vi "Beam Profiler.vi"(7 "Calling VI Ref":refnum<vi>) -> ()   [LabVIEW 2020]
uses:
  Hardware Configuration/Hardware Configuration Controls/Device Type.ctl
  Beam Profiler Controls/Beam Profiler Notifier Type.ctl
  Beam Profiler Controls/Beam Profiler Actions.ctl
  <vilib>/vision/Image Controls.llb/IMAQ Image.ctl
  <vilib>/Utility/miscctls.llb/LVPointTypeDef.ctl
  Device Library/Cameras/Camera Controls/Generic Camera ROI.ctl
  Beam Profiler Controls/Beam Profiler Fit Results.ctl
  Device Library/Cameras/Polymorphic Camera Messenger/Get Status.vi
  Device Library/Cameras/Polymorphic Camera Messenger/Abort.vi
  Device Library/Cameras/Polymorphic Camera Messenger/Set Exp Time.vi
  Device Library/Cameras/Polymorphic Camera Messenger/Get Exp Time.vi
  Device Library/Cameras/Polymorphic Camera Messenger/Set ROI.vi
  Device Library/Cameras/Polymorphic Camera Messenger/Live Preview.vi
  Device Library/Cameras/Polymorphic Camera Messenger/Quit.vi
  <vilib>/vision/NI_Vision_Development_Module.lvlib
panel:
  in  "Setup ROI":bool
  in  "ROI Active":bool
  out "Camera Connected":bool
  in  "Close Camera":bool
  in  "Quit":bool
  out "Y Pos (px)":dbl=1.0 format="%#_4g"
  out "X Pos (px)":dbl=1.0 format="%#_4g"
  out "Y FWHM (mm)":dbl=1.0 format="%#_4g"
  out "Y FWHM (px)":dbl=1.0 format="%#_4g"
  out "X FWHM (mm)":dbl=1.0 format="%#_4g"
  out "X FWHM (px)":dbl=1.0 format="%#_4g"
  in  "Cursor Visible":bool
  in  "Snap Cursor":bool
  in  "Color Map":T1(ring)=enum."Gray"
  out "Fit Image":dbl[][](graph)
  out "Camera Image":u16[][](graph)
  out "Error":bool
  in  "Live Preview":bool
  in  "Exposure Time (ms)":dbl=100.0
  in  "Camera Pixel Size (µm)":dbl=1.0
  in  "Fitting":bool
  in  "Fit Update Rate (ms)":u32=100
  in  "Binning (pixels)":i32=1 min=1 step=1
  in  "Profiler Camera":i32(ring) items=["IDS-Camera-Overview-3"]
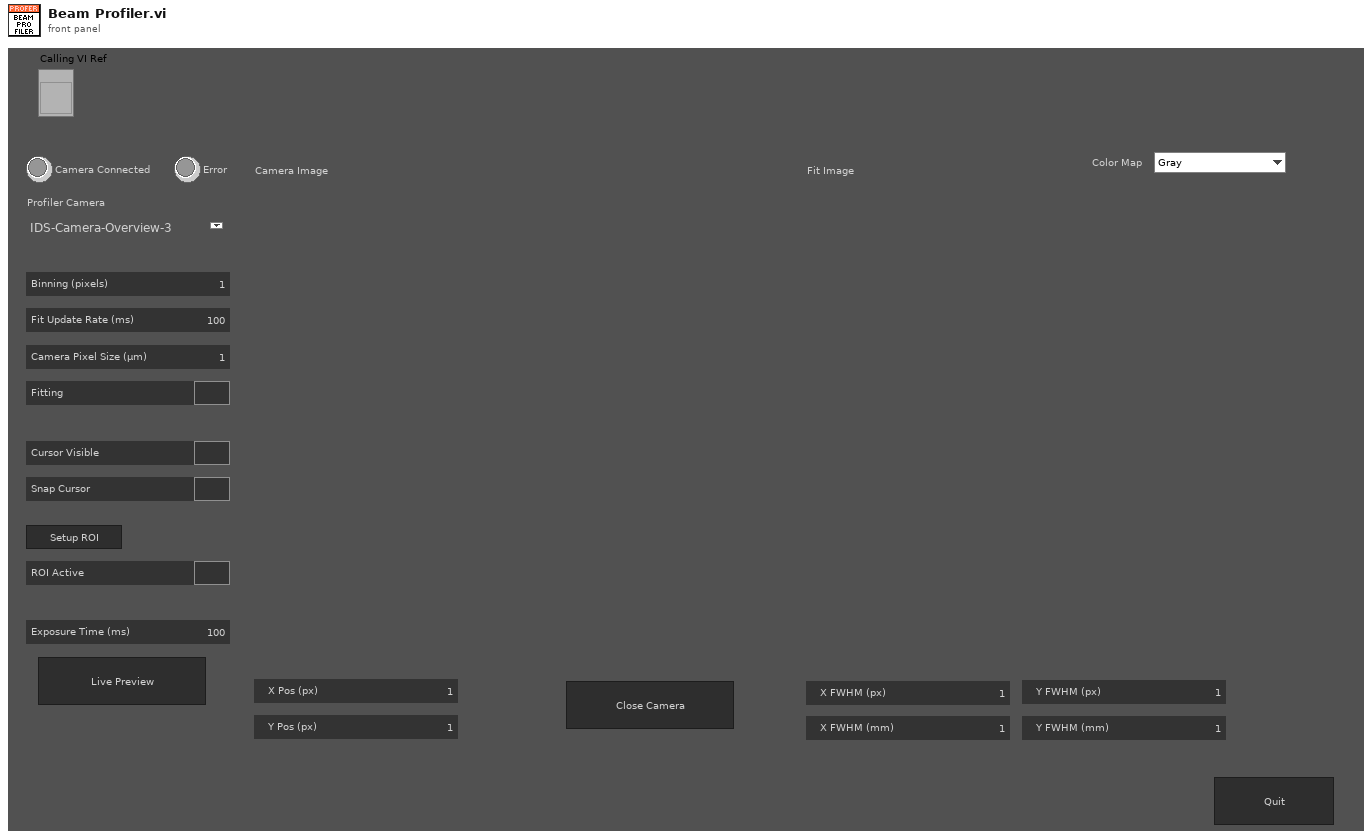
[diagram p1: front panel]
types:
  T1 = enum16{"Fire", "Gray", "Red", "Green", "Blue", "Cyan", "Magenta", "Yellow", "Red-White", "Green-White", "Blue-White", "Glow"}
  T2 = enum16{"Always On", "Always Off", "Off While Running"}
  T3 = typedef "LVPointTypeDef.ctl" = cluster{"Horizontal":i16, "Vertical":i16}
  T4 = typedef "Image Type" = u32
  T5 = typedef "IMAQ Image.ctl" = refnum<image>
  T6 = typedef "Beam Profiler Actions.ctl" = enum16{"Do Nothing", "Switch Camera", "Set Exp Time", "Setup ROI", "ROI Active", "Start Live", "Poll Image", "Stop Camera", "Quit"}
  T7 = typedef "Beam Profiler Notifier Type.ctl" = cluster{"Actions":T6, "Camera Notifier":string, "Pixel Size":dbl, "Binning":i32, "Fitting":bool, "Running?":bool, "Exp Time (ms)":dbl, "Image Ref":T5, "ROI Active":bool}
  T8 = typedef "Device Type.ctl" = enum16{"AOTF", "Camera", "Deformable Mirror", "Laser", "Microscope Base", "Shutter", "Stage", "Waveform", "FPGA", "Email", "Filter Wheel", "Spinning Disk"}
  T9 = typedef "Generic Camera ROI.ctl" = cluster{"H_Offset":u16, "V_Offset":u16, "H_Width":u16, "V_Width":u16}
  T10 = typedef "Beam Profiler Fit Results.ctl" = cluster{"X Position":dbl, "Y Position":dbl, "X FWHM (px)":dbl, "Y FWHM (px)":dbl, "X FWHM (mm)":dbl, "Y FWHM (mm)":dbl}
  T11 = enum8{"Enabled", "Disabled", "Disabled and Grayed Out"}
  T12 = typedef "LVRectTypeDef.ctl" = cluster{"Left":i16, "Top":i16, "Right":i16, "Bottom":i16}
  T13 = typedef "LVBoundsTypeDef.ctl" = cluster{"Width":u32, "Height":u32}
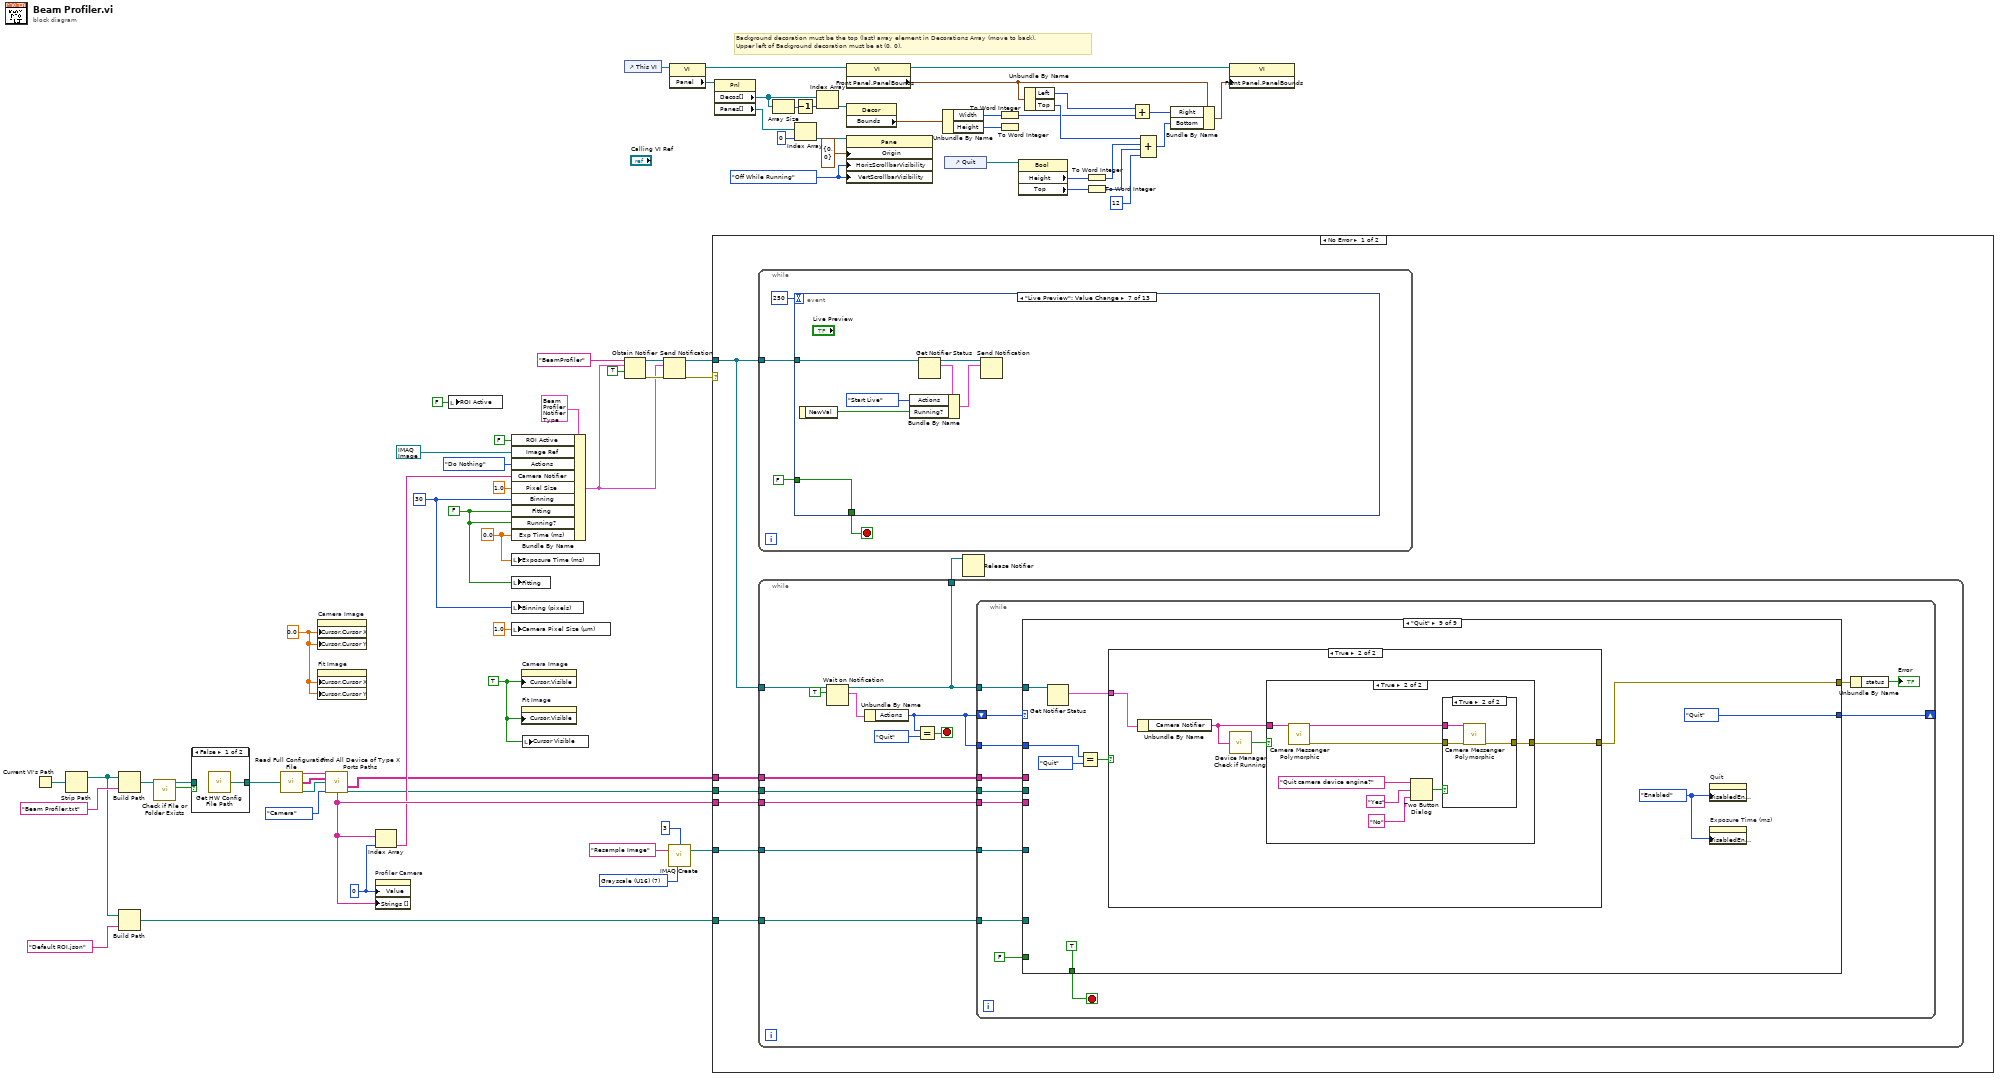
[diagram p0: block diagram]
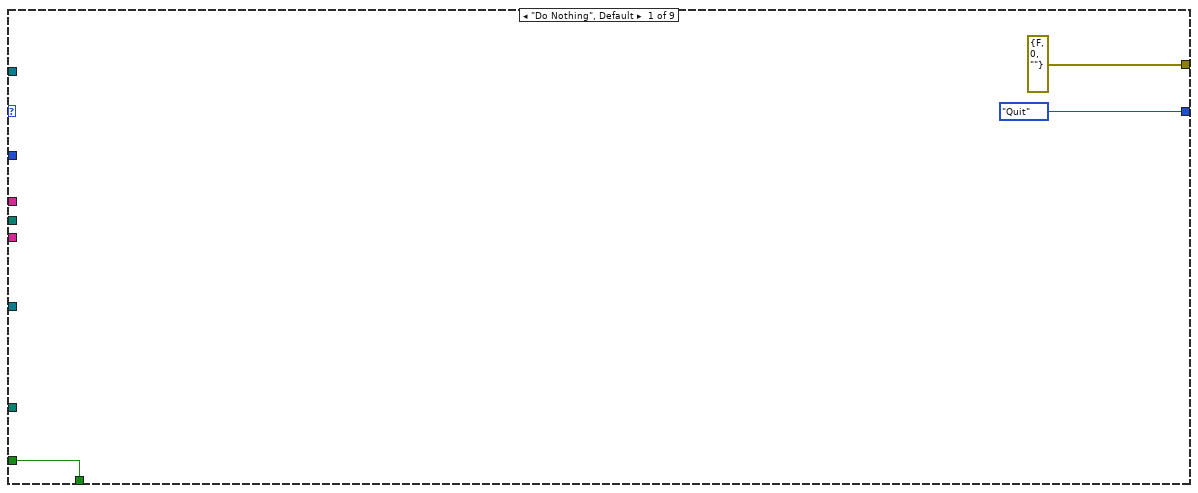
[diagram p3: hidden frame]
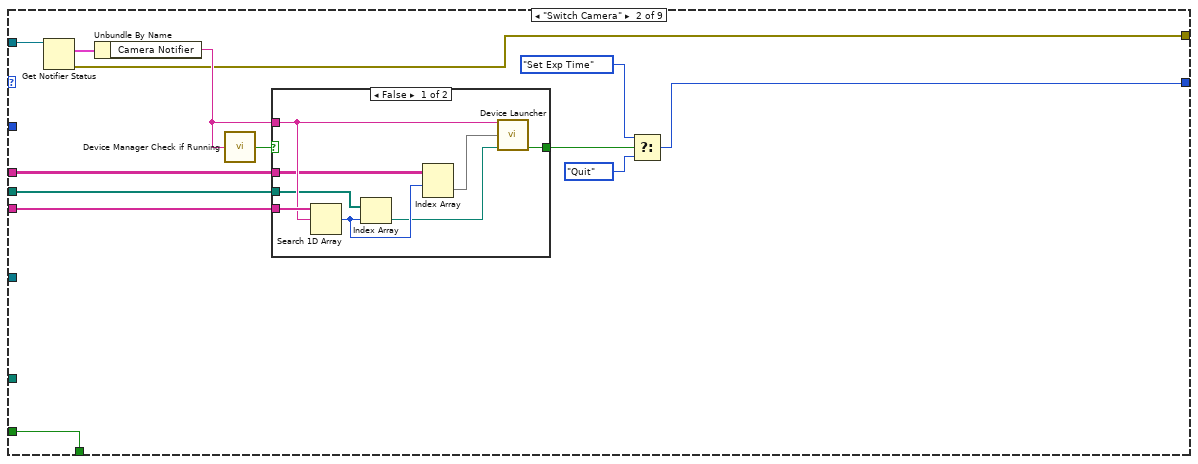
[diagram p4: hidden frame]
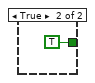
[diagram p5: hidden frame]
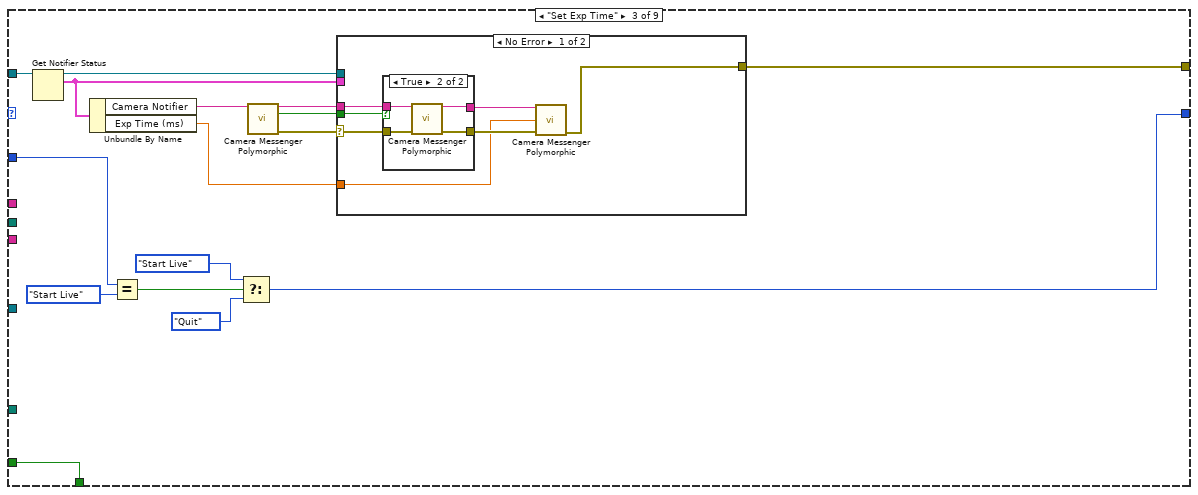
[diagram p6: hidden frame]
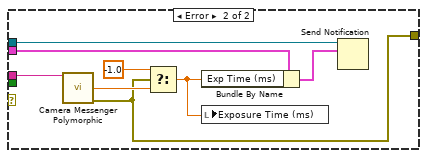
[diagram p8: hidden frame]
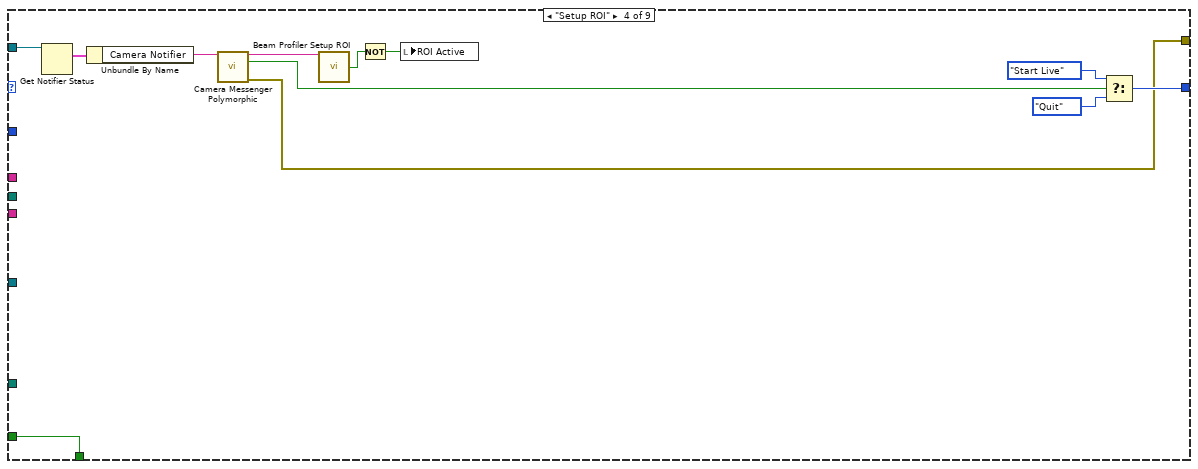
[diagram p9: hidden frame]
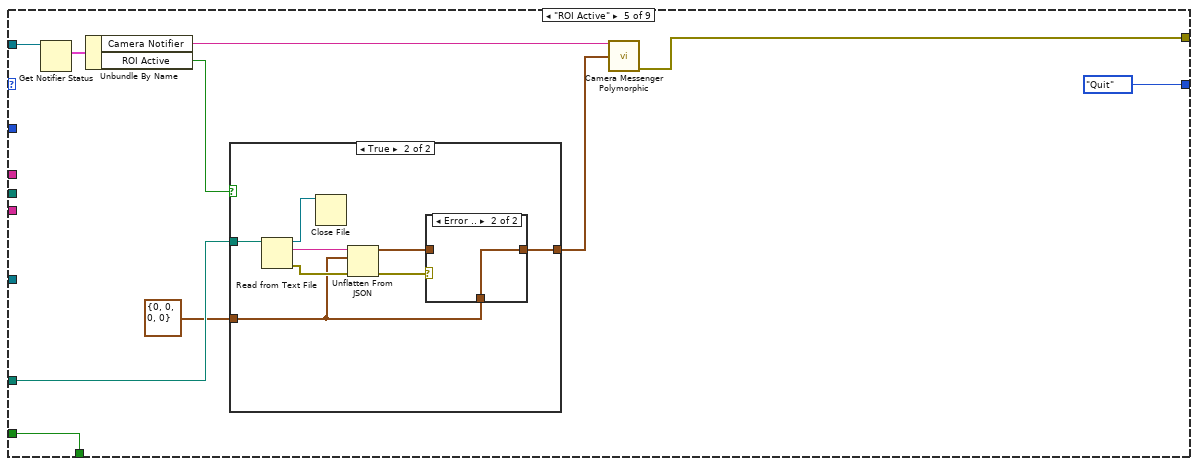
[diagram p10: hidden frame]
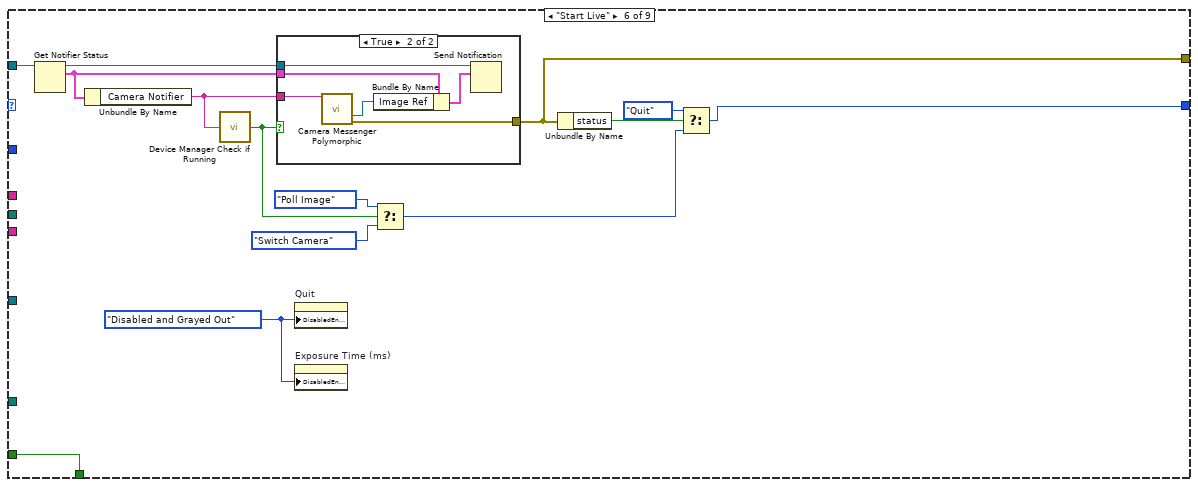
[diagram p13: hidden frame]
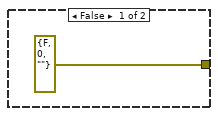
[diagram p14: hidden frame]
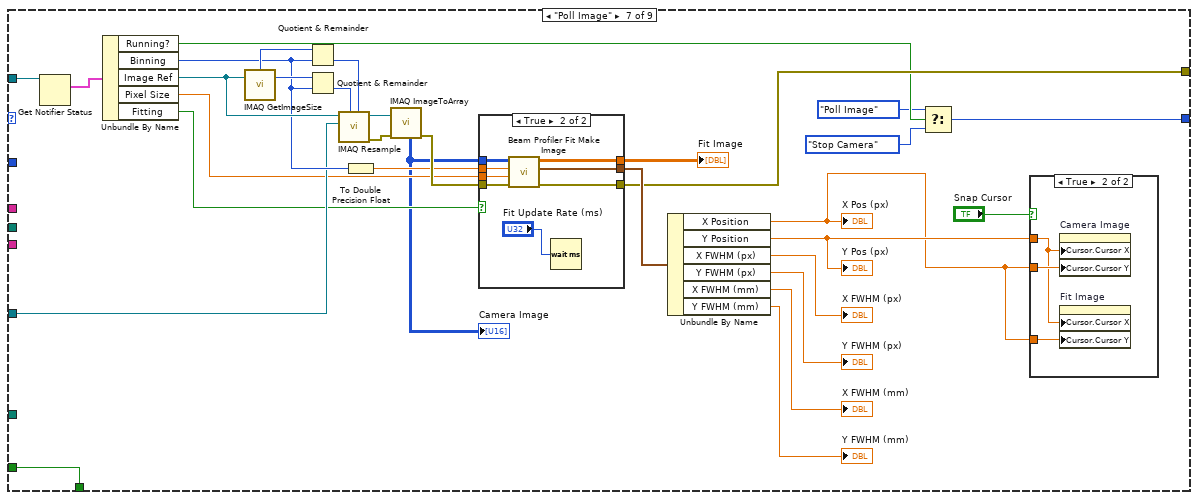
[diagram p15: hidden frame]
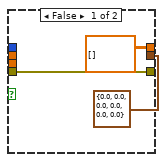
[diagram p17: hidden frame]
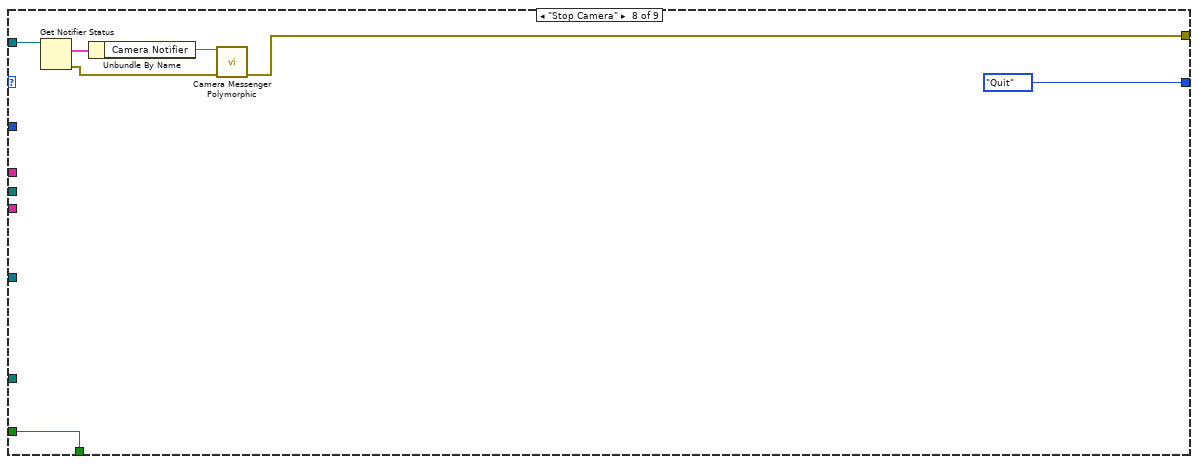
[diagram p18: hidden frame]
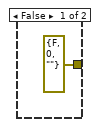
[diagram p19: hidden frame]
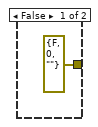
[diagram p20: hidden frame]
diagram:
  w16 = 0.0 ("Cursor.Cursor Position:Cursor X")
  w6 = TRUE ("Cursor.Visible")
  w29 = T2."Off While Running" ("Vertical Scrollbar Visibility")
  w52 = T4 7 items=["Grayscale (U8)", "Grayscale (I16)", "Grayscale (SGL)", "Complex (CSG)", "RGB (U32)", "HSL (U32)", "RGB (U64)", "Grayscale (U16)"] ("Image Type")
  w56 = 0.0 ("Exp Time (sec)")
  w59 = 30 ("Pixel Size")
  w60 = FALSE ("Fitting")
  w54 = 0
  # "Background decoration must be the top (last) array element in Decorations Array (move to back).\nUpper left of Background decoration must be at (0, 0)."
  n1 = Current VI's Path() -> (path=w15:path)
  n2 = Strip Path(path=w15) -> (stripped path=w8:path)  [unwired: 1 out]
  n3 = Build Path(base path=w8, name or relative path="Beam Profiler.txt") -> (appended path=w13:path)
  n4 = Build Path(base path=w8, name or relative path="Default ROI.json") -> (appended path=w7:path)
  n5 = call <vilib>:"Check if File or Folder Exists.vi"("path"=w13) -> ("file or folder exists?"=w12:bool, "dup path"=w11:path)  [unwired: 8 in, 1 out]
  n6 = case shown="False" w12 {
    tunnel: [w71 w72] -> w69
    tunnel: w11 -> [_ w72]
    frame False {
      n7 = call "Get HW Config File Path.vi"() -> ("File Path"=w71:path)  [unwired: 14 in, 1 out]
    }
    frame True {
    }
  }
  n8 = call "Read Full Configuration File.vi"("Config File Path"=w69) -> ("Unique Notifier Names"=w70:string[], "Device Port/ID/Channel Info"=w4:string[][], "Device Engine Paths"=w3:path[])  [unwired: 11 in, 1 out]
  n9 = property on="Camera Image" class="IntGraph (strict)"("Cursor.Cursor X"=w16, "Cursor.Cursor Y"=w16) -> ()  [unwired: 2 in, 2 out]
  n10 = property on="Fit Image" class="IntGraph (strict)"("Cursor.Cursor X"=w16, "Cursor.Cursor Y"=w16) -> ()  [unwired: 2 in, 2 out]
  n11 = call "Find All Device of Type X Ports Paths.vi"("Unique Notifier Names"=w70, "Device Port/ID/Channel Info"=w4, "Device Engine Paths"=w3, "Device Type"=Device_Type."Camera") -> ("All Ports"=w1:string[][], "All Devices"=w55:string[], "All Paths"=w2:path[])  [unwired: 8 in, 1 out]
  n12 = Index Array(array=w55, index=w54) -> (element=w17:string)
  n13 = property on="Profiler Camera" class="Ring (strict)"("Value"=w54, "Strings []"=w55) -> ()  [unwired: 2 in, 2 out]
  n14 = local write "ROI Active"(FALSE ("ROI Active")) -> ()
  n15 = Bundle By Name(cluster=T7 {"Actions"=enum."Do Nothing", "Camera Notifier"="", "Pixel Size"=0.0, "Binning"=0, "Fitting"=FALSE, "Running?"=FALSE, "Exp Time (ms)"=0.0, "Image Ref"=refnum, "ROI Active"=FALSE} ("Beam Profiler Notifier"), "ROI Active"=FALSE, "Image Ref"=T5 refnum, "Actions"=Beam_Profiler_Actions."Do Nothing", "Camera Notifier"=w17, "Pixel Size"=1.0, "Binning"=w59, "Fitting"=w60, "Running?"=w60, "Exp Time (ms)"=w56) -> (w61:T7)
  n16 = local write "Exposure Time (ms)"(w56) -> ()
  n17 = local write "Fitting"(w60) -> ()
  n18 = local write "Binning (pixels)"(w59) -> ()
  n19 = local write "Camera Pixel Size (µm)"(1.0 ("Camera Pixel Size (µm)")) -> ()
  n20 = property on="Camera Image" class="IntGraph (strict)"("Cursor.Visible"=w6) -> ()  [unwired: 2 in, 2 out]
  n21 = property on="Fit Image" class="IntGraph (strict)"("Cursor.Visible"=w6) -> ()  [unwired: 2 in, 2 out]
  n22 = local write "Cursor Visible"(w6) -> ()
  n23 = Obtain Notifier(name (unnamed)="BeamProfiler", notification data type=w61, create if not found? (T)=TRUE) -> (notifier out=w66:refnum<notifier>, error out=w65:errorcluster)  [unwired: 1 in, 1 out]
  n24 = control-ref of="This VI"() -> (w21:refnum<vi>)
  n25 = Send Notification(notification=w61, notifier=w66, error in (no error)=w65) -> (notifier out=w57:refnum<notifier>, error out=w58:errorcluster)
  n26 = call "IMAQ Create"("Border Size"=3, "Image Name"="Resample Image", "Image Type"=w52) -> ("New Image"=w49:T5)  [unwired: 2 in, 1 out]
  n27 = property class="VI"(reference=w21) -> (reference out=w30:refnum<vi>, "Panel"=w22:refnum<vi>)  [unwired: 1 in, 1 out]
  n28 = case shown="No Error" w58 {
    tunnel: w57 -> [w79 _]
    tunnel: w55 -> [w78 _]
    tunnel: w2 -> [w77 _]
    tunnel: w1 -> [w76 _]
    tunnel: w49 -> [w75 _]
    tunnel: w7 -> [w73 _]
    frame No Error {
      n29 = while {
        tunnel: w79 -> [w303]
        stop <- w301 stop-if-true
        n30 = event shown="[6] \"Live Preview\": Value Change" {
          selector: _ -> [_ _ _ _ _ _ _ _ _ _ _ _ _]
          dyn-events: _ -> [_ _ _ _ _ _ _ _ _ _ _ _ _]
          timeout: 250 -> [_ _ _ _ _ _ _ _ _ _ _ _ _]
          tunnel: w303 -> [w310 w319 w333 w338 w345 w352 w359 _ _ w382 w396 w415 w418]
          tunnel: FALSE -> [w311 w323 w336 w343 w350 w357 w364 w366 w369 w387 w406 w416 _]
          tunnel: [w311 w323 w336 w343 w350 w357 w364 w366 w369 w387 w406 w416 TRUE] -> w301
          event Timeout {
            n31 = event-data() -> ()  [unwired: 1 in, 3 out]
            n32 = Get Notifier Status(notifier=w310) -> (current notification=w309:T7)  [unwired: 1 in, 4 out]
            n33 = Unbundle By Name(w309) -> ("Camera Notifier"=w308:string)
            n34 = call "Device Manager Check if Running.vi"("Notifier Name"=w308) -> ("Running?"=w307:bool)  [unwired: 14 in]
            "Camera Connected" <- w307
            n35 = Select(t=T11."Enabled" ("Disabled"), s=w307, f=T11."Disabled and Grayed Out" ("Disabled")) -> (s? t:f=w304:T11)
            n36 = property on="Setup ROI" class="Bool"("DisabledEnum"=w304) -> ()  [unwired: 2 in, 2 out]
            n37 = property on="ROI Active" class="Bool (strict)"("DisabledEnum"=w304) -> ()  [unwired: 2 in, 2 out]
          }
          event "Profiler Camera": Value Change {
            n38 = event-data() -> ("NewVal"=w321:i32, "OldVal"=w314:i32)  [unwired: 1 in]
            n39 = property on="Profiler Camera" class="Ring (strict)"() -> ("Strings []"=w322:string[])  [unwired: 2 in, 2 out]
            n40 = Index Array(array=w322, index #1=w321, index #2=w314) -> (element #1=w317:string, element #2=w313:string)
            n41 = call-poly "Camera Messenger Polymorphic.vi"("Notifier Name"=w313) -> ("Error Out"=w312:errorcluster)  [unwired: 11 in, 3 out]
            n42 = Get Notifier Status(notifier=w319, error in (no error)=w312) -> (notifier out=w320:refnum<notifier>, current notification=w318:T7)  [unwired: 3 out]
            n43 = Bundle By Name(cluster=w318, "Actions"=Beam_Profiler_Actions."Switch Camera", "Camera Notifier"=w317) -> (w316:T7)
            n44 = Send Notification(notification=w316, notifier=w320) -> ()  [unwired: 1 in, 2 out]
          }
          event "Exposure Time (ms)": Value Change {
            n45 = event-data() -> ("NewVal"=w332:dbl)  [unwired: 1 in]
            n46 = Get Notifier Status(notifier=w333) -> (notifier out=w335:refnum<notifier>, current notification=w328:T7)  [unwired: 1 in, 3 out]
            n47 = Divide(x=w332, y=1000.0) -> (x/y=w330:dbl)
            n48 = Unbundle By Name(w328) -> ("Camera Notifier"=w329:string)
            n49 = call "Device Manager Check if Running.vi"("Notifier Name"=w329) -> ("Running?"=w327:bool)  [unwired: 14 in]
            n50 = Select(t=Beam_Profiler_Actions."Set Exp Time" ("Actions"), s=w327, f=Beam_Profiler_Actions."Switch Camera" ("Actions")) -> (s? t:f=w325:T6)
            n51 = Bundle By Name(cluster=w328, "Actions"=w325, "Exp Time (ms)"=w330) -> (w334:T7)
            n52 = Send Notification(notification=w334, notifier=w335) -> ()  [unwired: 1 in, 2 out]
          }
          event "Camera Pixel Size (µm)": Value Change {
            n53 = event-data() -> ("NewVal"=w337:dbl)  [unwired: 1 in]
            n54 = Get Notifier Status(notifier=w338) -> (notifier out=w342:refnum<notifier>, current notification=w341:T7)  [unwired: 1 in, 3 out]
            n55 = Bundle By Name(cluster=w341, "Actions"=Beam_Profiler_Actions."Do Nothing", "Pixel Size"=w337) -> (w340:T7)
            n56 = Send Notification(notification=w340, notifier=w342) -> ()  [unwired: 1 in, 2 out]
          }
          event "Binning (pixels)": Value Change {
            n57 = event-data() -> ("NewVal"=w344:i32)  [unwired: 1 in]
            n58 = Get Notifier Status(notifier=w345) -> (notifier out=w349:refnum<notifier>, current notification=w348:T7)  [unwired: 1 in, 3 out]
            n59 = Bundle By Name(cluster=w348, "Actions"=Beam_Profiler_Actions."Do Nothing", "Binning"=w344) -> (w347:T7)
            n60 = Send Notification(notification=w347, notifier=w349) -> ()  [unwired: 1 in, 2 out]
          }
          event "Fitting": Value Change {
            n61 = event-data() -> ("NewVal"=w351:bool)  [unwired: 1 in]
            n62 = Get Notifier Status(notifier=w352) -> (notifier out=w356:refnum<notifier>, current notification=w355:T7)  [unwired: 1 in, 3 out]
            n63 = Bundle By Name(cluster=w355, "Actions"=Beam_Profiler_Actions."Do Nothing", "Fitting"=w351) -> (w354:T7)
            n64 = Send Notification(notification=w354, notifier=w356) -> ()  [unwired: 1 in, 2 out]
          }
          event "Live Preview": Value Change {
            n65 = event-data() -> ("NewVal"=w358:bool)  [unwired: 1 in]
            n66 = Get Notifier Status(notifier=w359) -> (notifier out=w363:refnum<notifier>, current notification=w362:T7)  [unwired: 1 in, 3 out]
            n67 = Bundle By Name(cluster=w362, "Actions"=Beam_Profiler_Actions."Start Live", "Running?"=w358) -> (w361:T7)
            n68 = Send Notification(notification=w361, notifier=w363) -> ()  [unwired: 1 in, 2 out]
          }
          event "Cursor Visible": Value Change {
            n69 = event-data() -> ("NewVal"=w365:bool)  [unwired: 1 in]
            n70 = property on="Camera Image" class="IntGraph (strict)"("Cursor.Visible"=w365) -> ()  [unwired: 2 in, 2 out]
            n71 = property on="Fit Image" class="IntGraph (strict)"("Cursor.Visible"=w365) -> ()  [unwired: 2 in, 2 out]
          }
          event "Color Map": Value Change {
            n72 = event-data() -> ("NewVal"=w368:T1)  [unwired: 1 in]
            n73 = case shown="\"Fire\", Default" w368 {
              tunnel: [cluster{dbl, u32}[] [{0.0, 0}, {85.0, 16711680}, {108.0, 16729344}, {127.0, 16744192}, {132.0, 16747520}, {140.0, 16753920}, {157.0, 16766720}, {170.0, 16776960}, {245.0, 16777184}, {250.0, 16777200}, {255.0, 16777215}] ("Z Scale.Marker Values[]") cluster{dbl, u32}[] [{0.0, 0}, {255.0, 16777215}] ("Z Scale.Marker Values[]") cluster{dbl, u32}[] [{0.0, 0}, {255.0, 16711680}] ("Z Scale.Marker Values[]") cluster{dbl, u32}[] [{0.0, 0}, {255.0, 65280}] ("Z Scale.Marker Values[]") cluster{dbl, u32}[] [{0.0, 0}, {255.0, 255}] ("Z Scale.Marker Values[]") cluster{dbl, u32}[] [{0.0, 0}, {255.0, 65535}] ("Z Scale.Marker Values[]") cluster{dbl, u32}[] [{0.0, 0}, {255.0, 16711935}] ("Z Scale.Marker Values[]") cluster{dbl, u32}[] [{0.0, 0}, {255.0, 16776960}] ("Z Scale.Marker Values[]") cluster{dbl, u32}[] [{0.0, 0}, {170.0, 16711680}, {245.0, 16777184}, {250.0, 16777200}, {255.0, 16448250}] ("Z Scale.Marker Values[]") cluster{dbl, u32}[] [{0.0, 0}, {170.0, 65280}, {245.0, 16777184}, {250.0, 16777200}, {255.0, 16448250}] ("Z Scale.Marker Values[]") cluster{dbl, u32}[] [{0.0, 0}, {170.0, 255}, {245.0, 16777184}, {250.0, 16777200}, {255.0, 16448250}] ("Z Scale.Marker Values[]") cluster{dbl, u32}[] [{0.0, 0}, {1.0, 131072}, {2.0, 196608}, {3.0, 327680}, {4.0, 458752}, {5.0, 589824}, {6.0, 720896}, {7.0, 851971}, {8.0, 983043}, {9.0, 1114115}, {10.0, 1245187}, {11.0, 1376259}, {12.0, 1507331}, {13.0, 1638403}, {14.0, 1769475}, {15.0, 1769479}, {16.0, 2031623}, {17.0, 2162695}, {18.0, 2293767}, {19.0, 2424839}, {20.0, 2555911}, {21.0, 2686983}, {22.0, 2818055}, {23.0, 2949127}, {24.0, 3080203}, {25.0, 3211275}, {26.0, 3342347}, {27.0, 3473419}, {28.0, 3604491}, {29.0, 3735563}, {30.0, 3866635}, {31.0, 3867403}, {32.0, 4129547}, {33.0, 4260619}, {34.0, 4391691}, {35.0, 4522763}, {36.0, 4653839}, {37.0, 4784911}, {38.0, 4915983}, {39.0, 5178127}, {40.0, 5309199}, {41.0, 5440271}, {42.0, 5571343}, {43.0, 5702415}, {44.0, 5703439}, {45.0, 5965583}, {46.0, 6096655}, {47.0, 6227727}, {48.0, 6358799}, {49.0, 6489871}, {50.0, 6620943}, {51.0, 6752015}, {52.0, 6883087}, {53.0, 7015183}, {54.0, 7146255}, {55.0, 7277327}, {56.0, 7408399}, {57.0, 7539471}, {58.0, 7670543}, {59.0, 7801615}, {60.0, 8063759}, {61.0, 8194831}, {62.0, 8326927}, {63.0, 8457999}, {64.0, 8589075}, {65.0, 8720147}, {66.0, 8851219}, {67.0, 8982291}, {68.0, 9113363}, {69.0, 9114387}, {70.0, 9376531}, {71.0, 9507603}, {72.0, 9638675}, {73.0, 9769747}, {74.0, 9901843}, {75.0, 10032915}, {76.0, 10163987}, {77.0, 10229523}, {78.0, 10295059}, {79.0, 10427155}, {80.0, 10558227}, {81.0, 10689299}, {82.0, 10820371}, {83.0, 10886931}, {84.0, 10952467}, {85.0, 11083539}, {86.0, 11214611}, {87.0, 11215635}, {88.0, 11477779}, {89.0, 11543315}, {90.0, 11608851}, {91.0, 11740947}, {92.0, 11806483}, {93.0, 11872019}, {94.0, 12004115}, {95.0, 12135187}, {96.0, 12266259}, {97.0, 12267283}, {98.0, 12398355}, {99.0, 12529427}, {100.0, 12530451}, {101.0, 12595987}, {102.0, 12530451}, {103.0, 12793619}, {104.0, 12794131}, {105.0, 12794643}, {106.0, 13056787}, {107.0, 13057299}, {108.0, 13057811}, {109.0, 13188883}, {110.0, 13320979}, {111.0, 13386515}, {112.0, 13452563}, {113.0, 13584147}, {114.0, 13584659}, {115.0, 13585171}, {116.0, 13585683}, {117.0, 13717267}, {118.0, 13848339}, {119.0, 13849363}, {120.0, 13849875}, {121.0, 13850387}, {122.0, 13981459}, {123.0, 14113555}, {124.0, 14114067}, {125.0, 14114579}, {126.0, 14115091}, {127.0, 14246675}, {128.0, 14377747}, {129.0, 14378771}, {130.0, 14379283}, {131.0, 14379539}, {132.0, 14379795}, {133.0, 14380819}, {134.0, 14511891}, {135.0, 14643987}, {136.0, 14644503}, {137.0, 14645015}, {138.0, 14645527}, {139.0, 14646039}, {140.0, 14646551}, {141.0, 14778135}, {142.0, 14909207}, {143.0, 14910231}, {144.0, 14910747}, {145.0, 14911259}, {146.0, 14911771}, {147.0, 14912283}, {148.0, 14912797}, {149.0, 15044383}, {150.0, 15175455}, {151.0, 15175967}, {152.0, 15176479}, {153.0, 15176991}, {154.0, 15177507}, {155.0, 15178019}, {156.0, 15178531}, {157.0, 15310115}, {158.0, 15441701}, {159.0, 15441959}, {160.0, 15442215}, {161.0, 15442727}, {162.0, 15443243}, {163.0, 15443755}, {164.0, 15444269}, {165.0, 15444783}, {166.0, 15444783}, {167.0, 15576367}, {168.0, 15707953}, {169.0, 15708467}, {170.0, 15708979}, {171.0, 15708981}, {172.0, 15708983}, {173.0, 15710011}, {174.0, 15710523}, {175.0, 15711037}, {176.0, 15711039}, {177.0, 15711553}, {178.0, 15843139}, {179.0, 15974213}, {180.0, 15974215}, {181.0, 15974217}, {182.0, 15974219}, {183.0, 15975755}, {184.0, 15976271}, {185.0, 15976785}, {186.0, 15977299}, {187.0, 15977301}, {188.0, 15977815}, {189.0, 15978327}, {190.0, 15978331}, {191.0, 16109917}, {192.0, 16241503}, {193.0, 16241505}, {194.0, 16242019}, {195.0, 16242535}, {196.0, 16242537}, {197.0, 16242539}, {198.0, 16243563}, {199.0, 16243567}, {200.0, 16244081}, {201.0, 16244595}, {202.0, 16244599}, {203.0, 16244601}, {204.0, 16244603}, {205.0, 16245627}, {206.0, 16245631}, {207.0, 16245633}, {208.0, 16246147}, {209.0, 16246663}, {210.0, 16377735}, {211.0, 16508811}, {212.0, 16508815}, {213.0, 16509839}, {214.0, 16509843}, {215.0, 16509845}, {216.0, 16509847}, {217.0, 16510361}, {218.0, 16510875}, {219.0, 16510879}, {220.0, 16510881}, {221.0, 16510883}, {222.0, 16511399}, {223.0, 16511911}, {224.0, 16511915}, {225.0, 16511917}, {226.0, 16511919}, {227.0, 16511923}, {228.0, 16512437}, {229.0, 16512951}, {230.0, 16512955}, {231.0, 16512957}, {232.0, 16512959}, {233.0, 16512961}, {234.0, 16512963}, {235.0, 16512967}, {236.0, 16513481}, {237.0, 16513995}, {238.0, 16513999}, {239.0, 16514001}, {240.0, 16514003}, {241.0, 16514005}, {242.0, 16514007}, {243.0, 16514011}, {244.0, 16514013}, {245.0, 16514015}, {246.0, 16514019}, {247.0, 16514021}, {248.0, 16514023}, {249.0, 16514027}, {250.0, 16514029}, {251.0, 16514031}, {252.0, 16514035}, {253.0, 16514037}, {254.0, 16514039}, {255.0, 16514043}] ("Z Scale.Marker Values[]")] -> w367
              frame "Fire", Default {
                # "Fire"
              }
              frame "Gray" {
                # "Grayscale"
              }
              frame "Red" {
                # "Red"
              }
              frame "Green" {
                # "Green"
              }
              frame "Blue" {
                # "Blue"
              }
              frame "Cyan" {
                # "Cyan"
              }
              frame "Magenta" {
                # "Magenta"
              }
              frame "Yellow" {
                # "Yellow"
              }
              frame "Red-White" {
                # "Red-White"
              }
              frame "Green-White" {
                # "Green-White"
              }
              frame "Blue-White" {
                # "Blue-White"
              }
              frame "Glow" {
              }
            }
            n74 = property on="Camera Image" class="IntGraph (strict)"("ZScale.MarkerVals[]"=w367) -> ()  [unwired: 2 in, 2 out]
            n75 = property on="Fit Image" class="IntGraph (strict)"("ZScale.MarkerVals[]"=w367) -> ()  [unwired: 2 in, 2 out]
          }
          event "Setup ROI": Value Change {
            n76 = event-data() -> ()  [unwired: 1 in, 1 out]
            n77 = Get Notifier Status(notifier=w382) -> (notifier out=w386:refnum<notifier>, current notification=w385:T7)  [unwired: 1 in, 3 out]
            n78 = Bundle By Name(cluster=w385, "Actions"=Beam_Profiler_Actions."Setup ROI") -> (w384:T7)
            n79 = Send Notification(notification=w384, notifier=w386) -> ()  [unwired: 1 in, 2 out]
          }
          event "ROI Active": Value Change {
            n80 = event-data() -> ("NewVal"=w401:bool)  [unwired: 1 in]
            n81 = Get Notifier Status(notifier=w396) -> (notifier out=w398:refnum<notifier>, current notification=w399:T7, error out=w393:errorcluster)  [unwired: 1 in, 2 out]
            n82 = Bundle By Name(cluster=w399, "Actions"=Beam_Profiler_Actions."Do Nothing", "Running?"=FALSE) -> (w400:T7)
            n83 = Send Notification(notification=w400, notifier=w398, error in (no error)=w393) -> (notifier out=w394:refnum<notifier>, error out=w392:errorcluster)
            n84 = local write "Live Preview"(FALSE ("Live Preview")) -> ()
            n85 = while {
              tunnel: w394 -> [w412]
              tunnel: w392 -> [w411]
              tunnel: [w408] -> w391
              tunnel: [w407] -> w390
              stop <- w409 stop-if-true
              n86 = Get Notifier Status(notifier=w412, error in (no error)=w411) -> (notifier out=w408:refnum<notifier>, # waiting=w410:i32, error out=w407:errorcluster)  [unwired: 2 out]
              n87 = Greater Than 0?(x=w410) -> (x > 0?=w409:bool)
            }
            n88 = Get Notifier Status(notifier=w391, error in (no error)=w390) -> (notifier out=w405:refnum<notifier>, current notification=w404:T7, error out=w389:errorcluster)  [unwired: 2 out]
            n89 = Bundle By Name(cluster=w404, "Actions"=Beam_Profiler_Actions."ROI Active", "ROI Active"=w401) -> (w403:T7)
            n90 = Send Notification(notification=w403, notifier=w405, error in (no error)=w389) -> ()  [unwired: 2 out]
          }
          event "Close Camera": Value Change {
            n91 = event-data() -> ()  [unwired: 1 in, 1 out]
            n92 = Get Notifier Status(notifier=w415) -> (current notification=w414:T7)  [unwired: 1 in, 4 out]
            n93 = Unbundle By Name(w414) -> ("Camera Notifier"=w413:string)
            n94 = call-poly "Camera Messenger Polymorphic.vi"("Notifier Name"=w413) -> ()  [unwired: 13 in, 2 out]
          }
          event "Quit": Value Change {
            n95 = event-data() -> ()  [unwired: 1 in, 1 out]
            n96 = Get Notifier Status(notifier=w418) -> (notifier out=w422:refnum<notifier>, current notification=w421:T7)  [unwired: 1 in, 3 out]
            n97 = Bundle By Name(cluster=w421, "Actions"=Beam_Profiler_Actions."Quit") -> (w420:T7)
            n98 = Send Notification(notification=w420, notifier=w422) -> ()  [unwired: 1 in, 2 out]
          }
        }
      }
      n99 = while {
        tunnel: w79 -> [w91]
        tunnel: w78 -> [w87]
        tunnel: w77 -> [w86]
        tunnel: w76 -> [w85]
        tunnel: w75 -> [w83]
        tunnel: [w82] -> w74
        tunnel: w73 -> [w80]
        stop <- w88 stop-if-true
        n100 = Wait on Notification(notifier=w91, ignore previous (F)=TRUE) -> (notifier out=w82:refnum<notifier>, notification=w90:T7)  [unwired: 2 in, 2 out]
        n101 = Unbundle By Name(w90) -> ("Actions"=w84:T6)
        n102 = Equal?(x=w84, y=Beam_Profiler_Actions."Quit") -> (x = y?=w88:bool)
        n103 = while {
          tunnel: w82 -> [w103]
          tunnel: w87 -> [w100]
          tunnel: w86 -> [w99]
          tunnel: w85 -> [w98]
          shift-right: [w97] -> _
          shift-left: w84 -> [w104]
          tunnel: w84 -> [w96]
          tunnel: w83 -> [w95]
          tunnel: w80 -> [w92]
          stop <- w101 stop-if-true
          n104 = case shown="\"Quit\"" w104 {
            tunnel: w103 -> [_ w119 w145 w174 w187 w212 w250 w271 w277]
            tunnel: FALSE -> [w107 w120 w144 w178 w186 w213 w251 w270 _]
            tunnel: [w107 w120 w144 w178 w186 w213 w251 w270 TRUE] -> w101
            tunnel: w100 -> [_ w113 _ _ _ _ _ _ _]
            tunnel: w99 -> [_ w115 _ _ _ _ _ _ _]
            tunnel: w98 -> [_ w114 _ _ _ _ _ _ _]
            tunnel: [Beam_Profiler_Actions."Quit" ("f") w109 w133 w168 Beam_Profiler_Actions."Quit" ("f") w205 w225 Beam_Profiler_Actions."Quit" ("f") Beam_Profiler_Actions."Quit" ("f")] -> w97
            tunnel: [errorcluster {"status"=FALSE, "code"=0, "source"=""} ("Error Out") w108 w142 w167 w181 w208 w229 w267 w274] -> w93
            tunnel: w96 -> [_ _ w140 _ _ _ _ _ w278]
            tunnel: w95 -> [_ _ _ _ _ _ w240 _ _]
            tunnel: w92 -> [_ _ _ _ w184 _ _ _ _]
            frame "Do Nothing", Default {
            }
            frame "Switch Camera" {
              n105 = Get Notifier Status(notifier=w119) -> (current notification=w118:T7, error out=w108:errorcluster)  [unwired: 1 in, 3 out]
              n106 = Unbundle By Name(w118) -> ("Camera Notifier"=w116:string)
              n107 = call "Device Manager Check if Running.vi"("Notifier Name"=w116) -> ("Running?"=w117:bool)  [unwired: 14 in]
              n108 = case shown="False" w117 {
                tunnel: w116 -> [w127 _]
                tunnel: w115 -> [w125 _]
                tunnel: w114 -> [w126 _]
                tunnel: w113 -> [w128 _]
                tunnel: [w121 TRUE ("Running?")] -> w112
                frame False {
                  n109 = Search 1D Array(1D array=w128, element=w127) -> (index of element=w124:i32)  [unwired: 1 in]
                  n110 = Index Array(array=w125, index=w124) -> (element=w122:path)
                  n111 = Index Array(array=w126, index (row)=w124) -> (element=w123:string[])  [unwired: 1 in]
                  n112 = call "Device Launcher.vi"("Notifier Name"=w127, "Device Ports/IDs/Channels"=w123, "Device Engine Path"=w122) -> ("Running?"=w121:bool)  [unwired: 11 in, 1 out]
                }
                frame True {
                }
              }
              n113 = Select(t=Beam_Profiler_Actions."Set Exp Time" ("y"), s=w112, f=Beam_Profiler_Actions."Quit" ("y")) -> (s? t:f=w109:T6)
            }
            frame "Set Exp Time" {
              n114 = Get Notifier Status(notifier=w145) -> (notifier out=w136:refnum<notifier>, current notification=w135:T7)  [unwired: 1 in, 3 out]
              n115 = Unbundle By Name(w135) -> ("Camera Notifier"=w134:string, "Exp Time (ms)"=w143:dbl)
              n116 = Equal?(x=w140, y=Beam_Profiler_Actions."Start Live" ("x")) -> (x = y?=w139:bool)
              n117 = Select(t=Beam_Profiler_Actions."Start Live", s=w139, f=Beam_Profiler_Actions."Quit" ("y")) -> (s? t:f=w133:T6)
              n118 = call-poly "Camera Messenger Polymorphic.vi"("Notifier Name"=w134) -> ("Notifier Name DUP"=w131:string, "Running?"=w132:bool, "Error Out"=w130:errorcluster)  [unwired: 10 in, 2 out]
              n119 = case shown="No Error" w130 {
                selector: w130 -> [w146 _]
                tunnel: w132 -> [w152 _]
                tunnel: w131 -> [w151 w166]
                tunnel: w143 -> [w148 _]
                tunnel: [w147 w160] -> w142
                tunnel: w136 -> [_ w165]
                tunnel: w135 -> [_ w164]
                frame No Error {
                  n120 = case shown="True" w152 {
                    tunnel: w151 -> [w154 w158]
                    tunnel: w146 -> [w153 w157]
                    tunnel: [w154 w156] -> w150
                    tunnel: [w153 w155] -> w149
                    frame False {
                    }
                    frame True {
                      n121 = call-poly "Camera Messenger Polymorphic.vi"("Notifier Name"=w158, "Error In"=w157) -> ("Notifier Name DUP"=w156:string, "Error Out"=w155:errorcluster)  [unwired: 10 in, 2 out]
                    }
                  }
                  n122 = call-poly "Camera Messenger Polymorphic.vi"("Notifier Name"=w150, "Exp Time (s)"=w148, "Error In"=w149) -> ("Error Out"=w147:errorcluster)  [unwired: 9 in, 3 out]
                }
                frame Error {
                  n123 = call-poly "Camera Messenger Polymorphic.vi"("Notifier Name"=w166) -> ("Exp Time (s)"=w162:dbl, "Error Out"=w160:errorcluster)  [unwired: 12 in, 1 out]
                  n124 = Select(t=-1.0, s=w160, f=w162) -> (s? t:f=w159:dbl)
                  n125 = Bundle By Name(cluster=w164, "Exp Time (ms)"=w159) -> (w163:T7)
                  n126 = local write "Exposure Time (ms)"(w159) -> ()
                  n127 = Send Notification(notification=w163, notifier=w165) -> ()  [unwired: 1 in, 2 out]
                }
              }
            }
            frame "Setup ROI" {
              n128 = Get Notifier Status(notifier=w174) -> (current notification=w175:T7)  [unwired: 1 in, 4 out]
              n129 = Unbundle By Name(w175) -> ("Camera Notifier"=w173:string)
              n130 = call-poly "Camera Messenger Polymorphic.vi"("Notifier Name"=w173) -> ("Notifier Name DUP"=w172:string, "Running?"=w169:bool, "Error Out"=w167:errorcluster)  [unwired: 10 in, 2 out]
              n131 = call "Beam Profiler Setup ROI.vi"("Camera Notifier Name"=w172) -> ("Canceled?"=w177:bool)  [unwired: 14 in]
              n132 = Not(x=w177) -> (.not. x?=w176:bool)
              n133 = local write "ROI Active"(w176) -> ()
              n134 = Select(t=Beam_Profiler_Actions."Start Live" ("f"), s=w169, f=Beam_Profiler_Actions."Quit") -> (s? t:f=w168:T6)
            }
            frame "ROI Active" {
              n135 = Get Notifier Status(notifier=w187) -> (current notification=w188:T7)  [unwired: 1 in, 4 out]
              n136 = Unbundle By Name(w188) -> ("Camera Notifier"=w180:string, "ROI Active"=w185:bool)
              n137 = case shown="True" w185 {
                tunnel: w184 -> [_ w197]
                tunnel: [w189 w191] -> w182
                tunnel: T9 {"H_Offset"=0, "V_Offset"=0, "H_Width"=0, "V_Width"=0} ("General_Camera_ROI") -> [w189 w190]
                frame False {
                }
                frame True {
                  n138 = Read from Text File(file (use dialog)=w197) -> (refnum out=w195:refnum<file>, text=w196:string, error out=w194:errorcluster)  [unwired: 3 in, 1 out]
                  n139 = Close File(refnum=w195) -> ()  [unwired: 1 in, 2 out]
                  n140 = Unflatten From JSON(JSON string=w196, type and defaults=w190, error in (no error)=w194) -> (value=w192:T9, error out=w193:errorcluster)  [unwired: 4 in]
                  n141 = case shown="Error .." w193 {
                    tunnel: w192 -> [w198 _]
                    tunnel: [w198 w199] -> w191
                    tunnel: w190 -> [_ w199]
                    frame No Error {
                    }
                    frame Error {
                    }
                  }
                }
              }
              n142 = call-poly "Camera Messenger Polymorphic.vi"("Notifier Name"=w180, "Camera ROI"=w182) -> ("Error Out"=w181:errorcluster)  [unwired: 12 in, 1 out]
            }
            frame "Start Live" {
              w200 = T11."Disabled and Grayed Out" ("Disabled")
              n143 = Get Notifier Status(notifier=w212) -> (notifier out=w202:refnum<notifier>, current notification=w201:T7)  [unwired: 1 in, 3 out]
              n144 = Unbundle By Name(w201) -> ("Camera Notifier"=w209:string)
              n145 = call "Device Manager Check if Running.vi"("Notifier Name"=w209) -> ("Running?"=w210:bool)  [unwired: 14 in]
              n146 = case shown="True" w210 {
                tunnel: w209 -> [_ w220]
                tunnel: [errorcluster {"status"=FALSE, "code"=0, "source"=""} ("Error Out") w219] -> w208
                tunnel: w202 -> [_ w217]
                tunnel: w201 -> [_ w216]
                frame False {
                }
                frame True {
                  n147 = call-poly "Camera Messenger Polymorphic.vi"("Notifier Name"=w220) -> ("Image Ref"=w218:T5, "Error Out"=w219:errorcluster)  [unwired: 11 in, 2 out]
                  n148 = Bundle By Name(cluster=w216, "Image Ref"=w218) -> (w215:T7)
                  n149 = Send Notification(notification=w215, notifier=w217) -> ()  [unwired: 1 in, 2 out]
                }
              }
              n150 = property on="Quit" class="Bool"("DisabledEnum"=w200) -> ()  [unwired: 2 in, 2 out]
              n151 = property on="Exposure Time (ms)" class="DigNum (strict)"("DisabledEnum"=w200) -> ()  [unwired: 2 in, 2 out]
              n152 = Select(t=Beam_Profiler_Actions."Poll Image", s=w210, f=Beam_Profiler_Actions."Switch Camera" ("y")) -> (s? t:f=w207:T6)
              n153 = Unbundle By Name(w208) -> ("status"=w206:bool)
              n154 = Select(t=Beam_Profiler_Actions."Quit", s=w206, f=w207) -> (s? t:f=w205:T6)
            }
            frame "Poll Image" {
              n155 = Get Notifier Status(notifier=w250) -> (current notification=w249:T7)  [unwired: 1 in, 4 out]
              n156 = Unbundle By Name(w249) -> ("Running?"=w228:bool, "Binning"=w242:i32, "Image Ref"=w243:T5, "Pixel Size"=w237:dbl, "Fitting"=w236:bool)
              n157 = call "IMAQ GetImageSize"("Image"=w243) -> ("Y Resolution"=w246:i32, "X Resolution"=w245:i32)  [unwired: 3 in, 1 out]
              n158 = Quotient & Remainder(x=w245, y=w242) -> (floor(x/y)=w247:i32)  [unwired: 1 out]
              n159 = Quotient & Remainder(x=w246, y=w242) -> (floor(x/y)=w248:i32)  [unwired: 1 out]
              n160 = call "IMAQ Resample"("X Resolution"=w247, "Y Resolution"=w248, "Image Dst"=w240, "Image Src"=w243) -> ("error out"=w241:errorcluster, "Image Dst Out"=w244:T5)  [unwired: 6 in]
              n161 = To Double Precision Float(number=w242) -> (double precision float=w238:dbl)
              n162 = call "IMAQ ImageToArray"("error in (no error)"=w241, "Image"=w244) -> ("Image Pixels (U16)"=w221:u16[][], "error out"=w239:errorcluster)  [unwired: 2 in, 3 out]
              "Camera Image" <- w221
              n163 = case shown="True" w236 {
                tunnel: w221 -> [_ w265]
                tunnel: w239 -> [w256 w264]
                tunnel: w238 -> [_ w263]
                tunnel: w237 -> [_ w262]
                tunnel: [dbl[][] [] ("Fit Image") w261] -> w235
                tunnel: [w256 w260] -> w229
                tunnel: [T10 {"X Position"=0.0, "Y Position"=0.0, "X FWHM (px)"=0.0, "Y FWHM (px)"=0.0, "X FWHM (mm)"=0.0, "Y FWHM (mm)"=0.0} ("Fit Results") w259] -> w234
                frame False {
                }
                frame True {
                  n164 = call "Beam Profiler Fit Make Image.vi"("Error In"=w264, "Pixel Size (µm)"=w262, "Binning"=w263, "Image In (U16)"=w265) -> ("Error Out"=w260:errorcluster, "Fit Results"=w259:T10, "Fit Image"=w261:dbl[][])  [unwired: 5 in]
                  n165 = Wait (ms)(milliseconds to wait="Fit Update Rate (ms)") -> ()  [unwired: 1 out]
                }
              }
              "Fit Image" <- w235
              n166 = Unbundle By Name(w234) -> ("X Position"=w222:dbl, "Y Position"=w223:dbl, "X FWHM (px)"=→"X FWHM (px)":dbl, "Y FWHM (px)"=→"Y FWHM (px)":dbl, "X FWHM (mm)"=→"X FWHM (mm)":dbl, "Y FWHM (mm)"=→"Y FWHM (mm)":dbl)
              "X Pos (px)" <- w222
              "Y Pos (px)" <- w223
              n167 = Select(t=Beam_Profiler_Actions."Poll Image" ("y"), s=w228, f=Beam_Profiler_Actions."Stop Camera") -> (s? t:f=w225:T6)
              n168 = case shown="True" "Snap Cursor" {
                tunnel: w222 -> [_ w254]
                tunnel: w222 -> [_ w253]
                tunnel: w223 -> [_ w252]
                frame False {
                }
                frame True {
                  n169 = property on="Camera Image" class="IntGraph (strict)"("Cursor.Cursor X"=w252, "Cursor.Cursor Y"=w253) -> ()  [unwired: 2 in, 2 out]
                  n170 = property on="Fit Image" class="IntGraph (strict)"("Cursor.Cursor X"=w252, "Cursor.Cursor Y"=w254) -> ()  [unwired: 2 in, 2 out]
                }
              }
            }
            frame "Stop Camera" {
              n171 = Get Notifier Status(notifier=w271) -> (current notification=w272:T7, error out=w268:errorcluster)  [unwired: 1 in, 3 out]
              n172 = Unbundle By Name(w272) -> ("Camera Notifier"=w269:string)
              n173 = call-poly "Camera Messenger Polymorphic.vi"("Notifier Name"=w269, "Error In"=w268) -> ("Error Out"=w267:errorcluster)  [unwired: 10 in, 3 out]
            }
            frame "Quit" {
              w273 = T11."Enabled" ("Disabled")
              n174 = Get Notifier Status(notifier=w277) -> (current notification=w276:T7)  [unwired: 1 in, 4 out]
              n175 = Equal?(x=w278, y=Beam_Profiler_Actions."Quit") -> (x = y?=w275:bool)
              n176 = case shown="True" w275 {
                tunnel: w276 -> [_ w286]
                tunnel: [errorcluster {"status"=FALSE, "code"=0, "source"=""} ("error IO") w285] -> w274
                frame False {
                }
                frame True {
                  n177 = Unbundle By Name(w286) -> ("Camera Notifier"=w283:string)
                  n178 = call "Device Manager Check if Running.vi"("Notifier Name"=w283) -> ("Running?"=w284:bool)  [unwired: 14 in]
                  n179 = case shown="True" w284 {
                    tunnel: [errorcluster {"status"=FALSE, "code"=0, "source"=""} ("Error Out") w291] -> w285
                    tunnel: w283 -> [_ w290]
                    frame False {
                    }
                    frame True {
                      n180 = call-poly "Camera Messenger Polymorphic.vi"("Notifier Name"=w290) -> ("Notifier Name DUP"=w289:string, "Error Out"=w288:errorcluster)  [unwired: 11 in, 2 out]
                      n181 = Two Button Dialog(message="Quit camera device engine?", 1:"No" ("message"), 2:"Yes" ("message")) -> (T button?=w295:bool)
                      n182 = case shown="True" w295 {
                        tunnel: w289 -> [_ w299]
                        tunnel: w288 -> [w296 w298]
                        tunnel: [w296 w297] -> w291
                        frame False {
                        }
                        frame True {
                          n183 = call-poly "Camera Messenger Polymorphic.vi"("Notifier Name"=w299, "Error In"=w298) -> ("Error Out"=w297:errorcluster)  [unwired: 12 in, 1 out]
                        }
                      }
                    }
                  }
                }
              }
              n184 = property on="Quit" class="Bool"("DisabledEnum"=w273) -> ()  [unwired: 2 in, 2 out]
              n185 = property on="Exposure Time (ms)" class="DigNum (strict)"("DisabledEnum"=w273) -> ()  [unwired: 2 in, 2 out]
            }
          }
          n186 = Unbundle By Name(w93) -> ("status"=→"Error":bool)
        }
      }
      n187 = Release Notifier(notifier=w74) -> ()  [unwired: 2 in, 3 out]
    }
    frame Error {
    }
  }
  n188 = property class="Pnl"(reference=w22) -> ("Decos[]"=w20:refnum<vi>[], "Panes[]"=w26:refnum<vi>[])  [unwired: 1 in, 2 out]
  n189 = Array Size(array=w20) -> (size(s)=w18:i32)
  n190 = Decrement(x=w18) -> (x-1=w19:i32)
  n191 = Index Array(array=w26, index=0) -> (element=w25:refnum<vi>)
  n192 = Index Array(array=w20, index=w19) -> (element=w28:refnum<vi>)
  n193 = property class="VI"(reference=w30) -> (reference out=w32:refnum<vi>, "Front Panel.PanelBounds"=w33:T12)  [unwired: 1 in, 1 out]
  n194 = property class="Decor"(reference=w28) -> ("Bounds"=w31:T13)  [unwired: 1 in, 2 out]
  n195 = property class="Pane"(reference=w25, "Origin"=T3 {"Horizontal"=0, "Vertical"=0}, "HorizScrollbarVisibility"=w29, "VertScrollbarVisibility"=w29) -> ()  [unwired: 1 in, 2 out]
  n196 = Unbundle By Name(w31) -> ("Width"=w36:u32, "Height"=w39:u32)
  n197 = control-ref of="Quit"() -> (w23:refnum<vi>)
  n198 = To Word Integer(number=w36) -> (16bit integer=w38:i16)
  n199 = To Word Integer(number=w39) -> ()  [unwired: 1 out]
  n200 = property class="Bool"(reference=w23) -> ("Height"=w41:u32, "Top"=w42:i32)  [unwired: 1 in, 2 out]
  n201 = Unbundle By Name(w33) -> ("Left"=w35:i16, "Top"=w46:i16)
  n202 = To Word Integer(number=w41) -> (16bit integer=w44:i16)
  n203 = To Word Integer(number=w42) -> (16bit integer=w45:i16)
  n204 = Add(x=w35, y=w38) -> (x+y=w37:i16)
  n205 = Compound Arithmetic op=ADD(w46, w44, w45, i16 12 ("y")) -> (w40:i16)
  n206 = Bundle By Name(cluster=w33, "Right"=w37, "Bottom"=w40) -> (w34:T12)
  n207 = property class="VI"(reference=w32, "Front Panel.PanelBounds"=w34) -> ()  [unwired: 1 in, 2 out]
